vi "AGCxxx Query UnitS.vi"(8 "error in (no error)":errorcluster, 11 "AGCxxx VISA Cluster":T1={"VISA resource name"="", "VISA Timeout Value (1000 ms)"=1000, "Lock Timeout (1000 ms)"=1000, "MAX Channel (6)"=6}) -> (0 "error out":errorcluster, 1 "AGC Errno":i32, 2 "unit":enum16{"unknown", "mbar", "Pascal", "torr"}(ring), 3 "dup AGCxxx VISA Cluster":T1={"VISA resource name"="", "VISA Timeout Value (1000 ms)"=1000, "Lock Timeout (1000 ms)"=1000, "MAX Channel (6)"=6})   [LabVIEW 2014, in "AGCxxx - Driver.lvlib"]
doc: "Returns the current units setting for gauge units, as set in the CONFIG menu.\n\n1 = mbar\n2 = Pascal\n3 = torr\n\n\n\nCopyright (C) \nGesellschaft f. Schwerionenforschung, GSI\nPlanckstr. 1\n64291 Darmstadt\nGermany\n\nContact: http://www-wnt.gsi.de/labview\n H.Brand@gsi.de\n\nThis program is free software; you can redistribute it and/or\nmodify it under the terms of the GNU General Public License\nas published by the Free Software Foundation; either version 2\nof the License, or (at your option) any later version.\n\nThis program is distributed in the hope that it will be useful,\nbut WITHOUT ANY WARRANTY; without even the implied warranty of\nMERCHANTABILITY or FITNESS FOR A PARTICULAR PURPOSE. See the\nGNU General Public License for more details (http://www.gnu.org)."
uses:
  AGCxxx - Driver.lvlib
  AGCxxx VISA Control.ctl
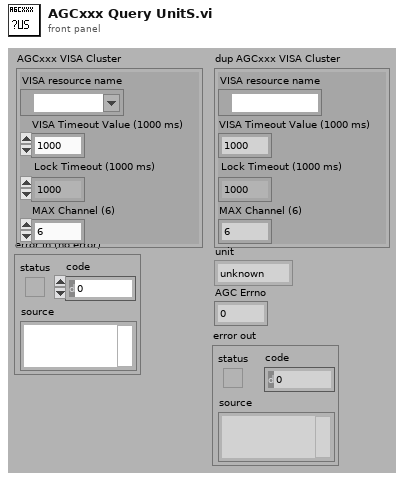
[diagram p1: front panel]
types:
  T1 = typedef "AGCxxx - Driver.lvlib/AGCxxx VISA Control.ctl" = cluster{"VISA resource name":refnum<visa-resource-name>, "VISA Timeout Value (1000 ms)":u32, "Lock Timeout (1000 ms)":u32, "MAX Channel (6)":i32}
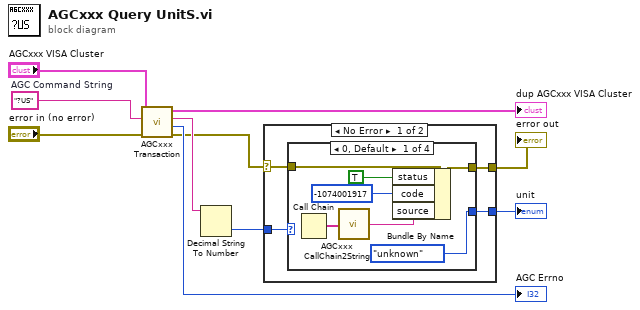
[diagram p0: block diagram]
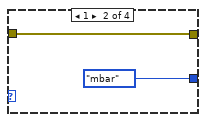
[diagram p2: hidden frame]
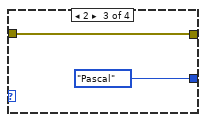
[diagram p3: hidden frame]
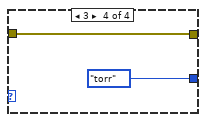
[diagram p4: hidden frame]
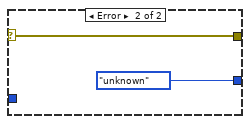
[diagram p5: hidden frame]
diagram:
  w8 = "?US"  # AGC Command String
  n1 = call "AGCxxx Transaction.vi"("error in (no error)"="error in (no error)", "AGC Command String"=w8, "AGCxxx VISA Cluster"="AGCxxx VISA Cluster") -> ("error out"=w2:errorcluster, "AGC Errno"=→"AGC Errno":i32, "AGC Response"=w9:string, "dup AGCxxx VISA Cluster"=→"dup AGCxxx VISA Cluster":T1)  [unwired: 4 in]
  n2 = Decimal String To Number(string=w9) -> (number=w10:i32)  [unwired: 2 in, 1 out]
  n3 = case shown="No Error" w2 {
    selector: w2 -> [w12 w28]
    tunnel: [w13 enum16{"unknown", "mbar", "Pascal", "torr"}."unknown"] -> w3
    tunnel: w10 -> [w14 _]
    tunnel: [w11 w28] -> w1
    frame No Error {
      n4 = case shown="0, Default" w14 {
        tunnel: [enum16{"unknown", "mbar", "Pascal", "torr"}."unknown" enum16{"unknown", "mbar", "Pascal", "torr"}."mbar" enum16{"unknown", "mbar", "Pascal", "torr"}."Pascal" enum16{"unknown", "mbar", "Pascal", "torr"}."torr"] -> w13
        tunnel: w12 -> [w16 w22 w24 w26]
        tunnel: [w15 w22 w24 w26] -> w11
        frame 0, Default {
          n5 = Call Chain() -> (call chain=w18:string[])
          n6 = call "AGCxxx CallChain2String.vi"("call chain"=w18) -> ("Call Chain String"=w17:string)
          n7 = Bundle By Name(cluster=w16, "status"=TRUE, "code"=-1074001917, "source"=w17) -> (w15:errorcluster)
        }
        frame 1 {
        }
        frame 2 {
        }
        frame 3 {
        }
      }
    }
    frame Error {
    }
  }
  "error out" <- w1
  "unit" <- w3
